vi "UI_Load_Spectrum_Modify.vi"() -> (2 "载荷谱初始行索引":i32, 3 "载荷谱修改":bool=TRUE)   [LabVIEW 2014]
uses:
  Terminal-Global-SetValues.vi
panel:
  in  "退出":bool
  in  "确认提交":bool
  in  "载荷谱表格":string[][](table)
  # "载荷谱修改"
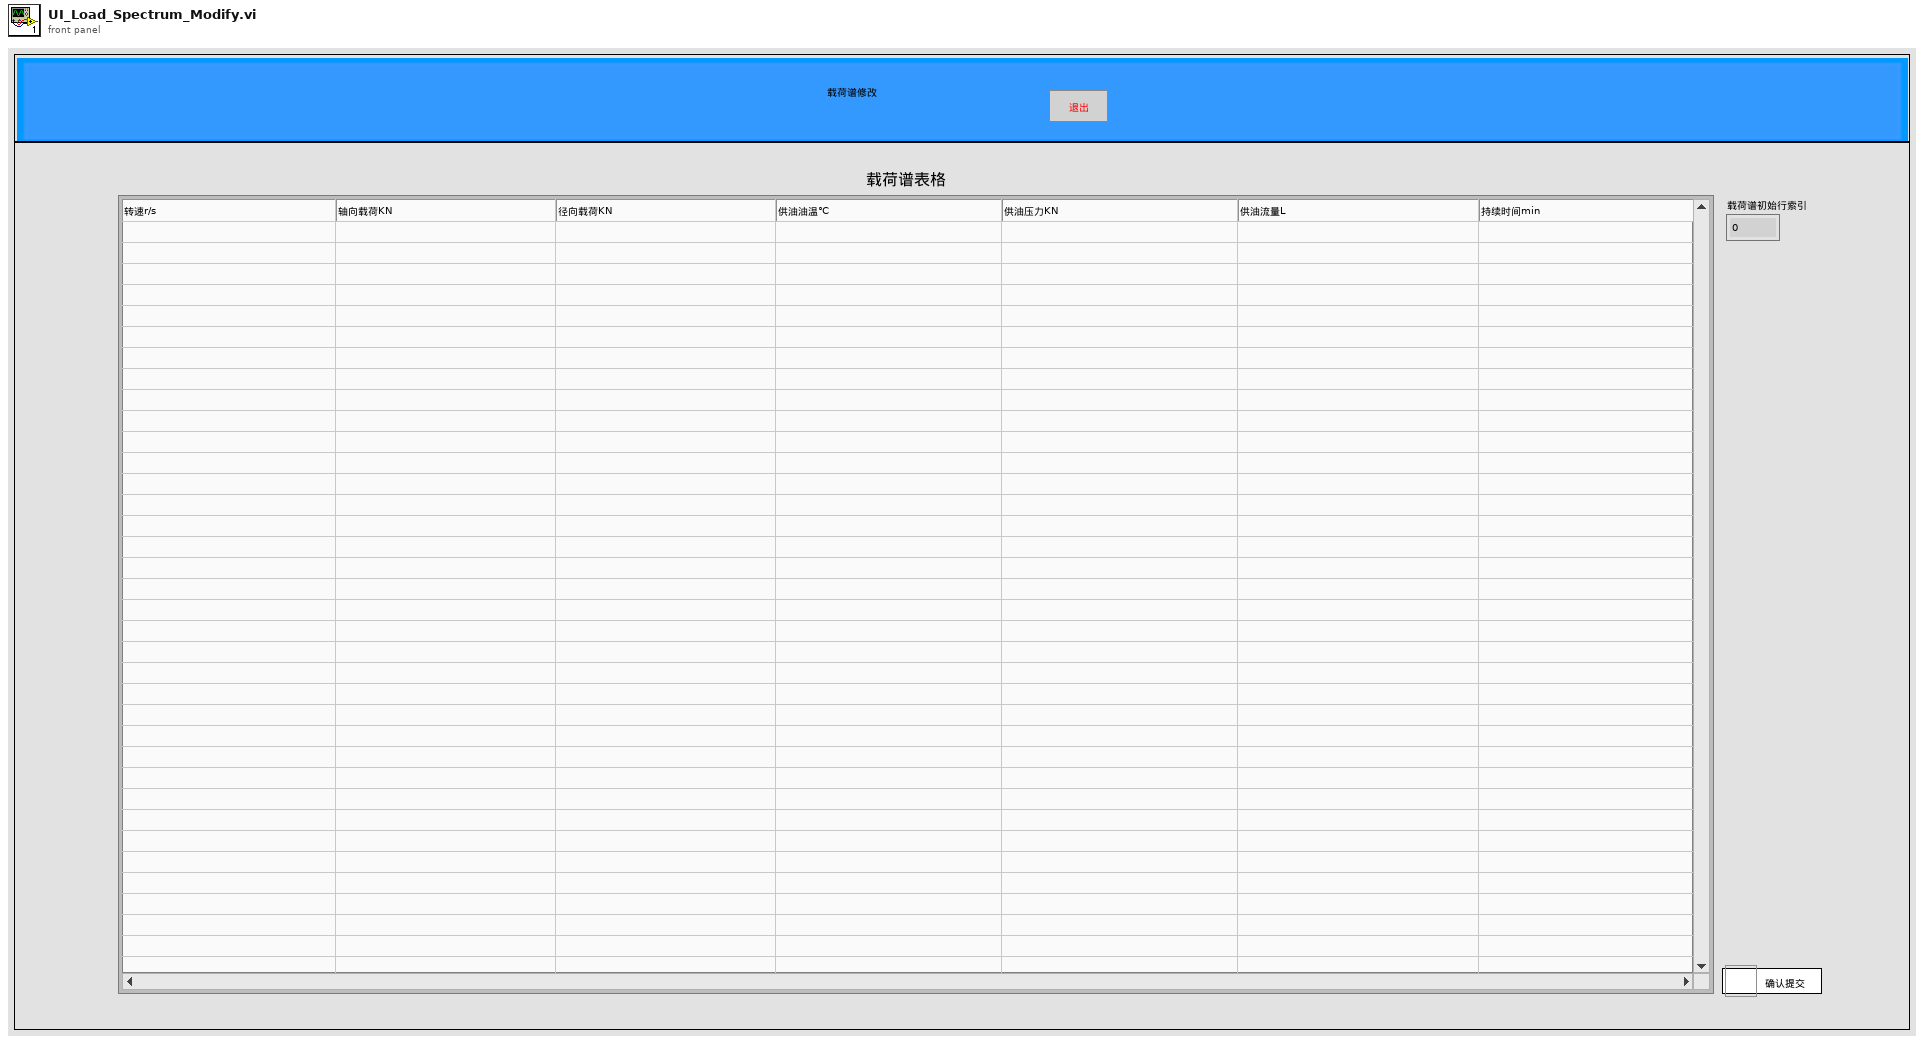
[diagram p1: front panel]
types:
  T1 = typedef "LVPoint32TypeDef.ctl" = cluster{"Horizontal":i32, "Vertical":i32}
  T2 = typedef "LVRowAndColumnTypeDef.ctl" = cluster{"Row":i32, "Column":i32}
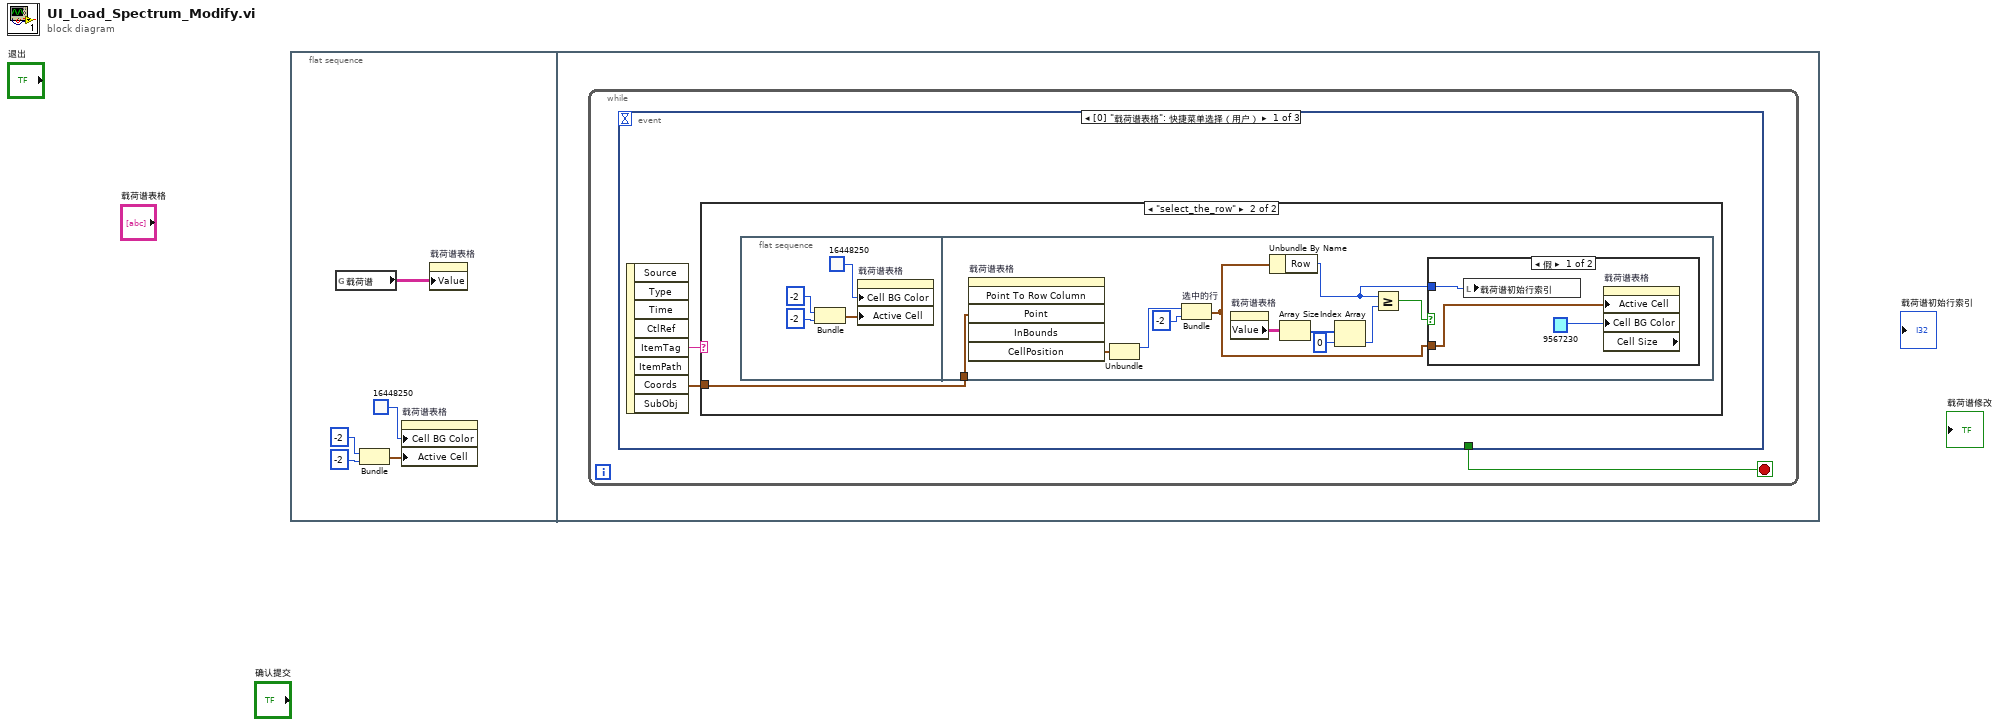
[diagram p0: block diagram]
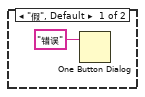
[diagram p2: hidden frame]
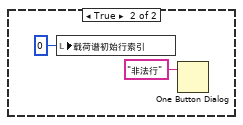
[diagram p3: hidden frame]
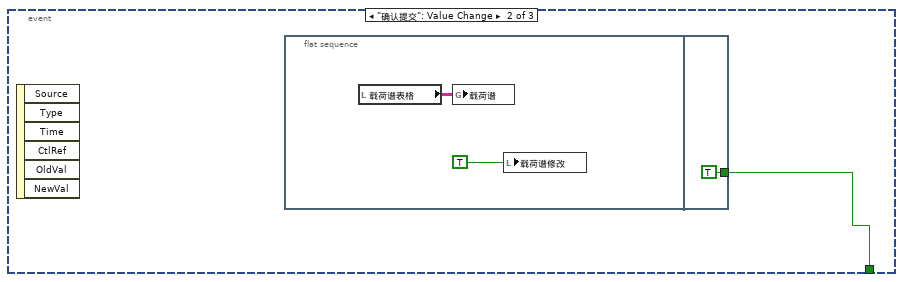
[diagram p4: hidden frame]
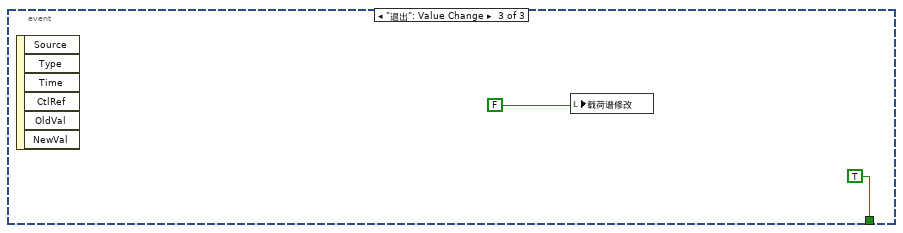
[diagram p5: hidden frame]
diagram:
  n1 = flat-sequence {
    frame #0 {
      n2 = global read "Terminal-Global-SetValues.vi" "载荷谱"() -> (w1:string[][])
      n3 = Bundle(-2, -2) -> (w4:cluster{i32, i32})  [unwired: 1 in]
      n4 = property on="载荷谱表格" class="Tbl (严格)"("Cell BG Color"=u32 16448250, "Active Cell"=w4) -> ()  [unwired: 2 in, 2 out]
      n5 = property on="载荷谱表格" class="Tbl (严格)"("Value"=w1) -> ()  [unwired: 2 in, 2 out]
    }
    frame #1 {
      n6 = while {
        stop <- w6 stop-if-true
        n7 = event shown="[0] \"载荷谱表格\": 快捷菜单选择（用户）" {
          selector: _ -> [_ _ _]
          dyn-events: _ -> [_ _ _]
          timeout: _ -> [_ _ _]
          tunnel: [_ w31 TRUE] -> w6
          event "载荷谱表格": Shortcut Menu Selection (User) {
            n8 = event-data() -> ("ItemTag"=w8:string, "Coords"=w7:T1)  [unwired: 1 in, 6 out]
            n9 = case shown="\"select_the_row\"" w8 {
              tunnel: w7 -> [_ w10]
              frame "假", Default {
                n10 = One Button Dialog(message="错误" ("消息")) -> ()  [unwired: 1 in, 1 out]
              }
              frame "select_the_row" {
                n11 = flat-sequence {
                  tunnel: w10 -> [w22]
                  frame #0 {
                    n12 = Bundle(-2, -2) -> (w12:cluster{i32, i32})  [unwired: 1 in]
                    n13 = property on="载荷谱表格" class="Tbl (严格)"("Cell BG Color"=u32 16448250, "Active Cell"=w12) -> ()  [unwired: 2 in, 2 out]
                  }
                  frame #1 {
                    n14 = invoke on="载荷谱表格" class="Tbl (严格)" method="Point To Row Column"("Point"=w22) -> ("CellPosition"=w23:T2)  [unwired: 5 in, 5 out]
                    n15 = Unbundle(w23) -> ("Row"=w24:i32)  [unwired: 1 out]
                    n16 = Bundle "选中的行"("Row"=w24, -2) -> (w20:cluster{"Row":i32, i32})  [unwired: 1 in]
                    n17 = property on="载荷谱表格" class="Tbl (严格)"() -> ("Value"=w16:string[][])  [unwired: 2 in, 2 out]
                    n18 = Unbundle By Name(w20) -> ("Row"=w19:i32)
                    n19 = Array Size(array=w16) -> (size(s)=w17:i32[])
                    n20 = Index Array(array=w17, index=0 ("索引")) -> (element=w15:i32)
                    n21 = Greater Or Equal?(x=w19, y=w15) -> (x >= y?=w21:bool)
                    n22 = case shown="假" w21 {
                      tunnel: w20 -> [w27 _]
                      tunnel: w19 -> [w26 _]
                      frame False {
                        n23 = local write "载荷谱初始行索引"(w26) -> ()
                        n24 = property on="载荷谱表格" class="Tbl (严格)" props=["Active Cell", "Cell BG Color", "Cell Size"]("Active Cell"=w27, "Cell BG Color"=u32 9567230) -> ()  [unwired: 2 in, 3 out]
                      }
                      frame True {
                        n25 = local write "载荷谱初始行索引"(0 ("载荷谱初始行索引")) -> ()
                        n26 = One Button Dialog(message="非法行" ("消息")) -> ()  [unwired: 1 in, 1 out]
                      }
                    }
                  }
                }
              }
            }
          }
          event "确认提交": Value Change {
            n27 = event-data() -> ()  [unwired: 1 in, 6 out]
            n28 = flat-sequence {
              tunnel: [TRUE] -> w31
              frame #0 {
                n29 = local read "载荷谱表格"() -> (w33:string[][])
                n30 = global write "Terminal-Global-SetValues.vi" "载荷谱"(w33) -> ()
                n31 = local write "载荷谱修改"(TRUE) -> ()
              }
              frame #1 {
              }
            }
          }
          event "退出": Value Change {
            n32 = event-data() -> ()  [unwired: 1 in, 6 out]
            n33 = local write "载荷谱修改"(FALSE) -> ()
          }
        }
      }
    }
  }
